vi "Send Message.vi"(7 "Priority Message? (F)":bool, 10 "error in (no error)":errorcluster, 11 "Message":T1={"Source"="", "Destination"="", "Time Stamp"=timestamp(0 s since 1904-01-01), "Command"="", "Data"=variant(string "")}) -> (2 "error out":errorcluster)   [LabVIEW 2020, in "Dynamic Reentrant.lvlib"]
doc: "Send a message to the named queue based on the Destination field of the Message typedef. If no queue with the name contained in Destination exists, a new queue is NOT created and error 1100 is thrown."
uses:
  Dynamic Reentrant.lvlib
  Type Defs/Message.ctl
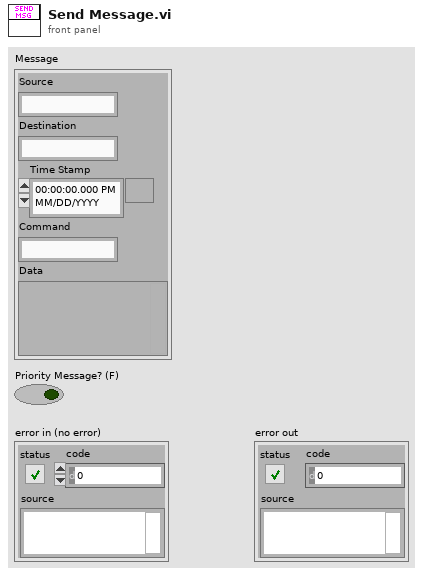
[diagram p1: front panel]
types:
  T1 = typedef "Dynamic Reentrant.lvlib/Message.ctl" = cluster{"Source":string, "Destination":string, "Time Stamp":timestamp, "Command":string, "Data":variant}
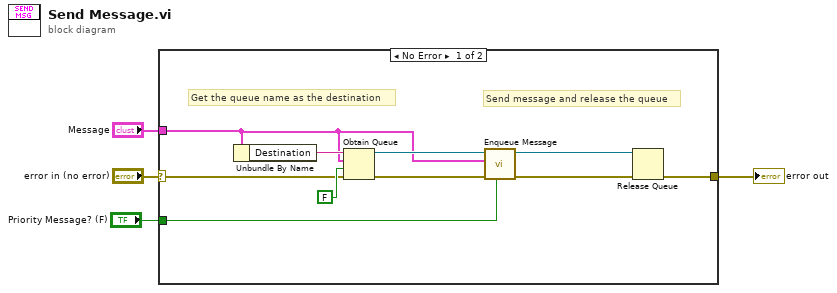
[diagram p0: block diagram]
diagram:
  n1 = case shown="No Error" "error in (no error)" {
    selector: "error in (no error)" -> [w11 w15]
    tunnel: [w14 w15] -> w4
    tunnel: "Message" -> [w8 _]
    tunnel: "Priority Message? (F)" -> [w5 _]
    frame No Error {
      # "Send message and release the queue"
      # "Get the queue name as the destination"
      n2 = Unbundle By Name(w8) -> ("Destination"=w13:string)
      n3 = Obtain Queue(name (unnamed)=w13, element data type=w8, create if not found? (T)=FALSE, error in (no error)=w11) -> (queue out=w10:refnum<queue>, error out=w7:errorcluster)  [unwired: 1 in, 1 out]
      n4 = call "Enqueue Message.vi"("Priority Message? (F)"=w5, "error in (no error)"=w7, "Message"=w8, "Listening Queue"=w10) -> ("error out"=w6:errorcluster, "queue out"=w9:refnum<queue>)  [unwired: 6 in]
      n5 = Release Queue(queue=w9, error in (no error)=w6) -> (error out=w14:errorcluster)  [unwired: 1 in, 2 out]
    }
    frame Error {
    }
  }
  "error out" <- w4
